vi "REC_ThermalCAM_simple.vi"() -> ()   [LabVIEW 2018]
doc: "To use this browser, you can type in a URL in the location field and then click on the Go button. You can also use the Back, Forward, Reload and Search buttons. This VI also has a runtime menu which is included in the library. When you run the VI, you will have File Menu and a History Menu. The file menu contains the same functionality that the buttons can do and the History menu contains a History of all the pages that you have visited in a given session.\n\nThe Invoke Node and Property Node functions are used to control the operation of the web browser. For more information on the Microsoft Web Browser Control, see Microsoft's web site (try http://support.microsoft.com/support/kb/articles/q165/2/12.asp)."
panel:
  in  "Stop Button":bool
  in  "Search":bool
  in  "Go":bool
  in  "Reload":bool
  in  "Back":bool
  in  "Forward":bool
  in  "URL :":string="192.168.1.65"
  in  "SHDocVw.IWebBrowser2":refnum<k7>(container)
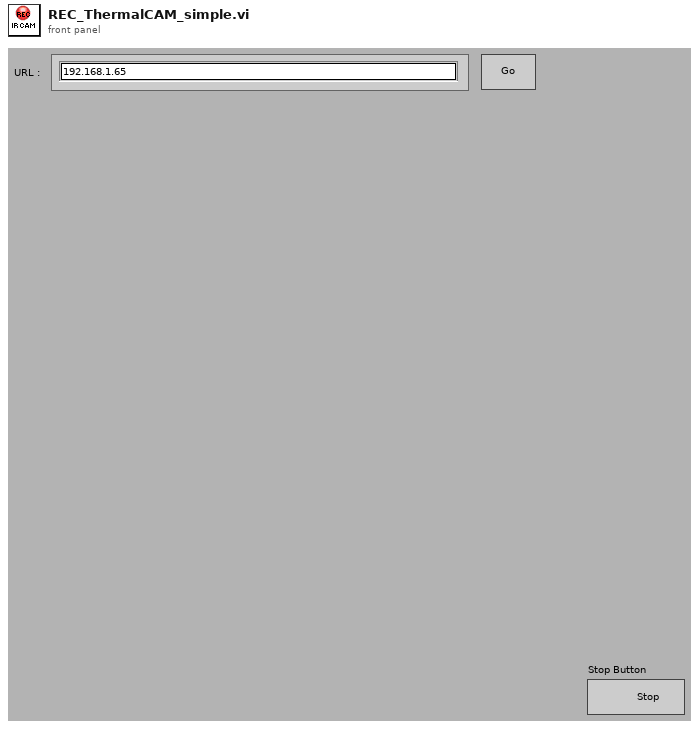
[diagram p1: front panel]
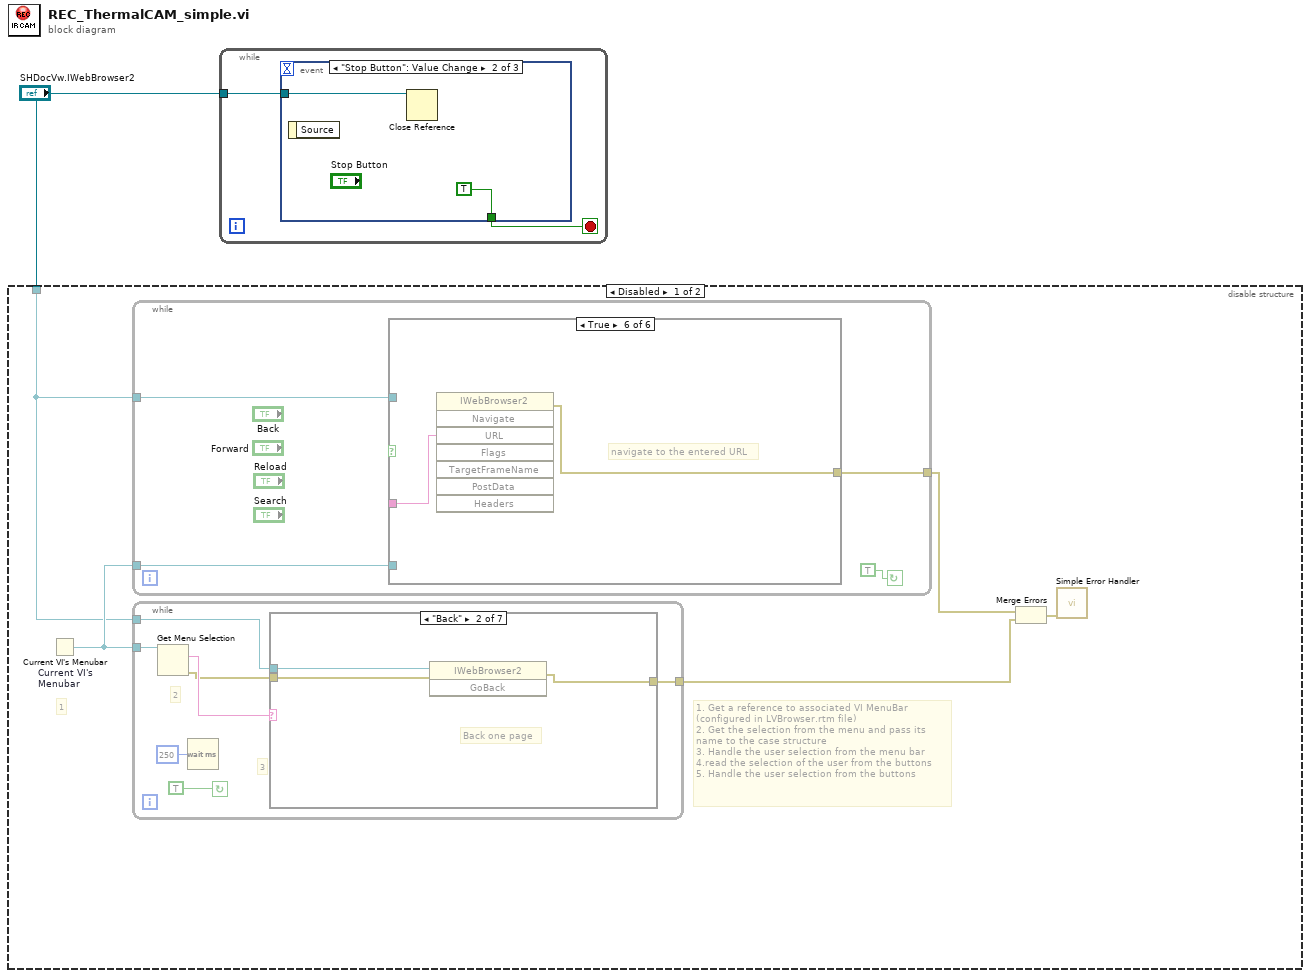
[diagram p0: block diagram]
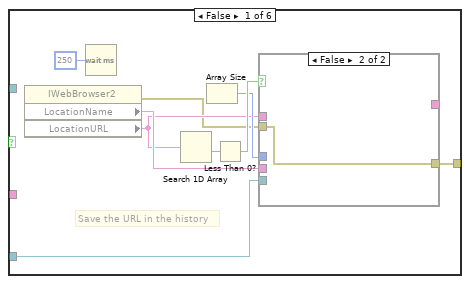
[diagram p2: hidden frame]
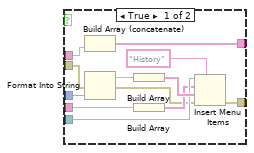
[diagram p3: hidden frame]
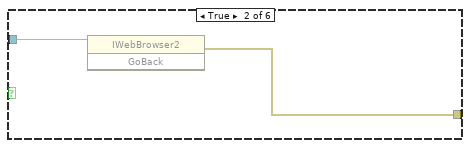
[diagram p4: hidden frame]
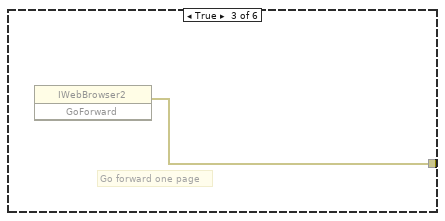
[diagram p5: hidden frame]
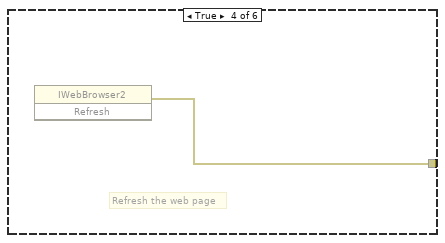
[diagram p6: hidden frame]
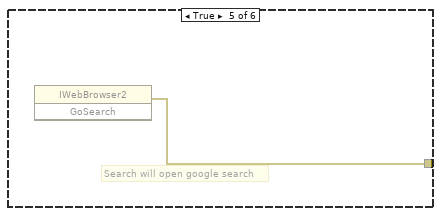
[diagram p7: hidden frame]
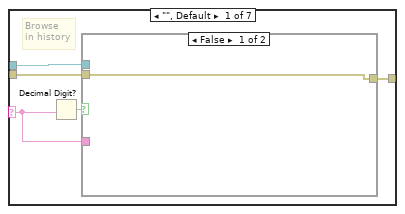
[diagram p8: hidden frame]
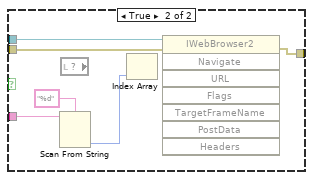
[diagram p9: hidden frame]
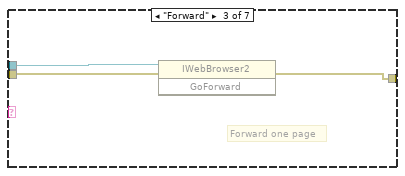
[diagram p10: hidden frame]
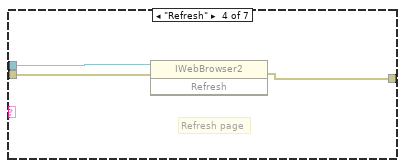
[diagram p11: hidden frame]
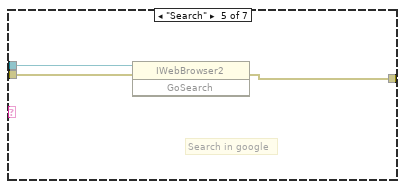
[diagram p12: hidden frame]
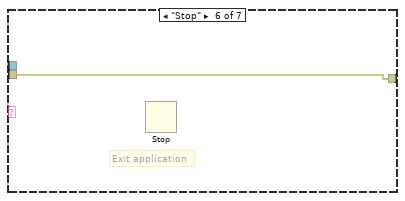
[diagram p13: hidden frame]
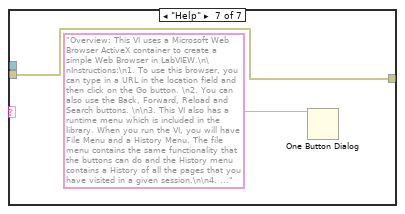
[diagram p14: hidden frame]
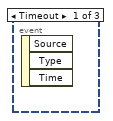
[diagram p16: hidden frame]
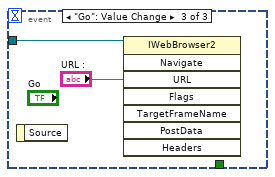
[diagram p17: hidden frame]
diagram:
  n1 = disable-structure shown="Disabled" {
    disable-tunnel: "SHDocVw.IWebBrowser2" -> [w2 _]
    frame Disabled {
      # "1. Get a reference to associated VI MenuBar \n(configured in LVBrowser.rtm file)\n2. Get the selection from the menu and pass its \nname to the case structure\n3. Handle the user selection from the menu bar\n4.read the selection of the user from the buttons\n5. Handle the user selection from the buttons"
      # "1"
      n2 = Current VI's Menubar "Current VI's \nMenubar"() -> (w6:refnum<k9>)
      n3 = while {
        tunnel: w6 -> [w9]
        tunnel: [w8] -> w5
        tunnel: w2 -> [w7]
        stop <- TRUE continue-if-true
        n4 = case shown="True" {
          selector: _ -> [_ _ _ _ _ _]
          tunnel: _ -> [_ _ _ _ _ w39]
          tunnel: w9 -> [w13 _ _ _ _ _]
          tunnel: [w12 w34 w35 w36 w37 w38] -> w8
          tunnel: w7 -> [_ w33 _ _ _ _]
          frame False {
            # "Save the URL in the history"
            n5 = property class="IWebBrowser2"() -> (error out=w11:errorcluster, "LocationName"=w19:string, "LocationURL"=w14:string)  [unwired: 2 in, 1 out]
            n6 = Wait (ms)(milliseconds to wait=u32 250 ("millisecond multiple")) -> ()  [unwired: 1 out]
            n7 = Search 1D Array(element=w14) -> (index of element=w18:i32)  [unwired: 2 in]
            n8 = Array Size() -> (size(s)=w16:i32)  [unwired: 1 in]
            n9 = Less Than 0?(x=w18) -> (x < 0?=w17:bool)
            n10 = case shown="False" w17 {
              tunnel: w13 -> [w28 _]
              tunnel: w19 -> [w26 _]
              tunnel: w14 -> [w23 _]
              tunnel: w16 -> [w24 _]
              tunnel: [w25 _] -> _
              tunnel: [w21 w32] -> w12
              tunnel: w11 -> [w20 w32]
              frame True {
                n11 = Build Array (concatenate)(w23) -> (w25:string[])  [unwired: 1 in]
                n12 = Format Into String(error in=w20, w24) -> (resulting string=w31:string, error out=w22:errorcluster)  [unwired: 2 in]
                n13 = Build Array(w31) -> (w30:string[])
                n14 = Build Array(w26) -> (w27:string[])
                n15 = Insert Menu Items(5:"History" ("menu tag"), 6:w22, 7:w30, 8:w27, 9:w28) -> (0:w21:errorcluster)  [unwired: 1 in, 2 out]
              }
              frame False {
              }
            }
          }
          frame True {
            n16 = invoke class="IWebBrowser2" method="GoBack"(reference=w33) -> (error out=w34:errorcluster)  [unwired: 2 in, 2 out]
          }
          frame True {
            # "Go forward one page"
            n17 = invoke class="IWebBrowser2" method="GoForward"() -> (error out=w35:errorcluster)  [unwired: 3 in, 2 out]
          }
          frame True {
            # "Refresh the web page"
            n18 = invoke class="IWebBrowser2" method="Refresh"() -> (error out=w36:errorcluster)  [unwired: 3 in, 2 out]
          }
          frame True {
            # "Search will open google search"
            n19 = invoke class="IWebBrowser2" method="GoSearch"() -> (error out=w37:errorcluster)  [unwired: 3 in, 2 out]
          }
          frame True {
            # "navigate to the entered URL"
            n20 = invoke class="IWebBrowser2" method="Navigate"("URL"=w39) -> (error out=w38:errorcluster)  [unwired: 7 in, 7 out]
          }
        }
      }
      n21 = while {
        tunnel: w6 -> [w45]
        tunnel: w2 -> [w43]
        tunnel: [w40] -> w4
        stop <- TRUE continue-if-true
        # "3"
        # "2"
        n22 = Get Menu Selection(0:w45) -> (6:w44:string, 8:w41:errorcluster)  [unwired: 3 in, 3 out]
        n23 = Wait (ms)(milliseconds to wait=u32 250 ("millisecond multiple")) -> ()  [unwired: 1 out]
        n24 = case shown="\"Back\"" w44 {
          selector: w44 -> [w49 _ _ _ _ _ _]
          tunnel: w43 -> [w51 w61 w64 w67 w70 _ _]
          tunnel: w41 -> [w48 w60 w63 w66 w69 w71 w72]
          tunnel: [w47 w59 w62 w65 w68 w71 w72] -> w40
          frame "", Default {
            # "Browse\nin history"
            n25 = Decimal Digit?(1:w49) -> (0:w50:bool)
            n26 = case shown="False" w50 {
              tunnel: w51 -> [_ w58]
              tunnel: w49 -> [_ w56]
              tunnel: w48 -> [w52 w54]
              tunnel: [w52 w53] -> w47
              frame False {
              }
              frame True {
                n27 = Scan From String(format string="%d", input string=w56) -> (output 1=w55:i32)  [unwired: 3 in, 3 out]
                n28 = local read item#-1() -> ()  [unwired: 1 out]
                n29 = Index Array(index=w55) -> ()  [unwired: 1 in, 1 out]
                n30 = invoke class="IWebBrowser2" method="Navigate"(reference=w58, error in=w54) -> (error out=w53:errorcluster)  [unwired: 6 in, 7 out]
              }
            }
          }
          frame "Back" {
            # "Back one page"
            n31 = invoke class="IWebBrowser2" method="GoBack"(reference=w61, error in=w60) -> (error out=w59:errorcluster)  [unwired: 1 in, 2 out]
          }
          frame "Forward" {
            # "Forward one page"
            n32 = invoke class="IWebBrowser2" method="GoForward"(reference=w64, error in=w63) -> (error out=w62:errorcluster)  [unwired: 1 in, 2 out]
          }
          frame "Refresh" {
            # "Refresh page"
            n33 = invoke class="IWebBrowser2" method="Refresh"(reference=w67, error in=w66) -> (error out=w65:errorcluster)  [unwired: 1 in, 2 out]
          }
          frame "Search" {
            # "Search in google"
            n34 = invoke class="IWebBrowser2" method="GoSearch"(reference=w70, error in=w69) -> (error out=w68:errorcluster)  [unwired: 1 in, 2 out]
          }
          frame "Stop" {
            # "Exit application"
            n35 = Stop() -> ()  [unwired: 1 in]
          }
          frame "Help" {
            n36 = One Button Dialog(message="Overview: This VI uses a Microsoft Web Browser ActiveX container to create a simple Web Browser in LabVIEW.\n\nInstructions:\n1. To use this browser, you can type in a URL in the location field and then click on the Go button. \n2. You can also use the Back, Forward, Reload and Search buttons. \n\n3. This VI also has a runtime menu which is included in the library. When you run the VI, you will have File Menu and a History Menu. The file menu contains the same functionality that the buttons can do and the History menu contains a History of all the pages that you have visited in a given session.\n\n4. To Stop Execution, Click on File>> Stop") -> ()  [unwired: 1 in, 1 out]
          }
        }
      }
      n37 = Merge Errors(w5, w4) -> (w3:errorcluster)
      n38 = call <vilib>:"Simple Error Handler.vi"("error in (no error)"=w3) -> ()  [unwired: 4 in, 5 out]
    }
    frame Enabled {
    }
  }
  n39 = while {
    tunnel: "SHDocVw.IWebBrowser2" -> [w74]
    stop <- w75 stop-if-true
    n40 = event shown="[1] \"Stop Button\": Value Change" {
      selector: _ -> [_ _ _]
      dyn-events: _ -> [_ _ _]
      timeout: _ -> [_ _ _]
      tunnel: [_ TRUE _] -> w75
      tunnel: w74 -> [_ w76 w78]
      event Timeout {
        n41 = event-data() -> ()  [unwired: 1 in, 3 out]
      }
      event "Stop Button": Value Change {
        n42 = event-data() -> ()  [unwired: 1 in, 1 out]
        n43 = Close Reference(reference=w76) -> ()  [unwired: 1 in, 1 out]
      }
      event "Go": Value Change {
        n44 = event-data() -> ()  [unwired: 1 in, 1 out]
        n45 = invoke class="IWebBrowser2" method="Navigate"(reference=w78, "URL"="URL :") -> ()  [unwired: 6 in, 8 out]
      }
    }
  }
